vi "List.vi"(11 "Circular Buffer in":refnum<class "Circular Buffer.lvclass">) -> (0 "Decryption List":i64[](array[numeric]), 1 "Shift List":i64[](array[numeric]), 2 "Node List":refnum<data-value>[](array[refnum]), 3 "Circular Buffer out":refnum<class "Circular Buffer.lvclass">)   [LabVIEW 2021, in "d20.lvlib" / "Circular Buffer.lvclass"]
uses:
  Circular Buffer.lvclass
  INode/INode.lvclass
  Circular Buffer.lvclass/Circular Buffer.ctl
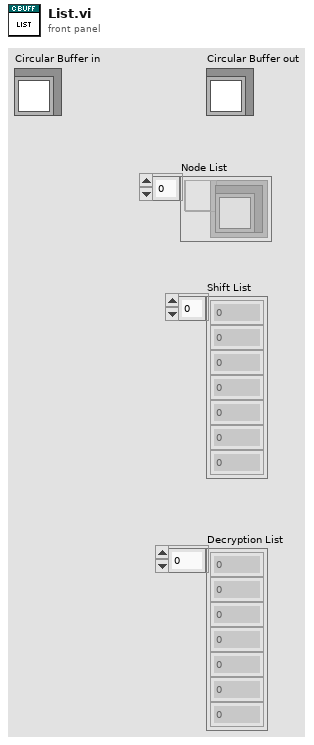
[diagram p1: front panel]
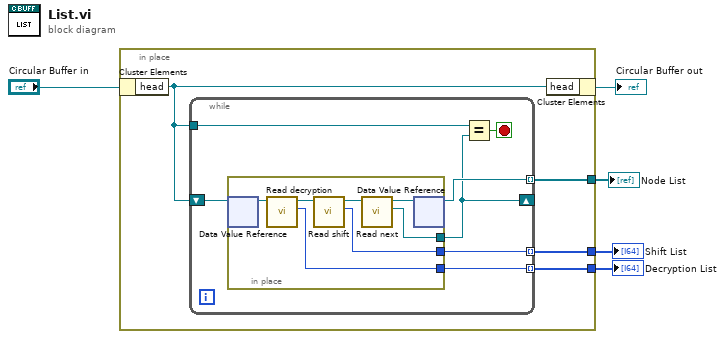
[diagram p0: block diagram]
diagram:
  n1 = in-place {
    in-place-border: [w9] -> w3
    in-place-border: [w8] -> w2
    in-place-border: [w6] -> w1
    n2 = in-place-cluster #1("Circular Buffer in") -> ("head"=w7:refnum<data-value>)
    n3 = while {
      shift-right: [w13] -> _
      shift-left: w7 -> [w12]
      tunnel: [w16] -> w9 mode=indexing
      tunnel: [w14] -> w8 mode=indexing
      tunnel: w7 -> [w11]
      tunnel: [w10] -> w6 mode=indexing
      stop <- w15 stop-if-true
      n4 = in-place {
        in-place-border: [w21] -> w16
        in-place-border: [w23] -> w13
        in-place-border: [w19] -> w10
        n5 = in-place-dvr #2(w12) -> (w18:refnum<class "INode.lvclass">)  [unwired: 1 out]
        n6 = call-dynamic "Read decryption.vi"("INode in"=w18) -> ("decryption"=w19:i64, "INode out"=w20:refnum<class "INode.lvclass">)  [unwired: 9 in]
        n7 = call-dynamic "Read shift.vi"("Node in"=w20) -> ("shift"=w21:i64, "Node out"=w22:refnum<class "INode.lvclass">)  [unwired: 9 in]
        n8 = call-dynamic "Read next.vi"("Node in"=w22) -> ("next"=w23:refnum<data-value>, "Node out"=w17:refnum<class "INode.lvclass">)  [unwired: 9 in]
        n9 = in-place-dvr #2(w17) -> (w14:refnum<data-value>)  [unwired: 1 out]
      }
      n10 = Equal?(x=w11, y=w13) -> (x = y?=w15:bool)
    }
    n11 = in-place-cluster #1("head"=w7) -> (→"Circular Buffer out":refnum<class "Circular Buffer.lvclass">)
  }
  "Shift List" <- w3
  "Decryption List" <- w1
  "Node List" <- w2
